vi "fireEventSendRefs.vi"(8 "error in (no error)":errorcluster, 10 "objectRefsMain":T1, 11 "sendRefs":refnum<user-event>) -> (0 "error out":errorcluster)   [LabVIEW 2017, in "User Event - Stop.lvlib"]
doc: "Send the Stop event to stop the Event Handling Loop."
uses:
  User Event - Stop.lvlib
  Controls/objectRefsMain.ctl
  sendRefs.ctl
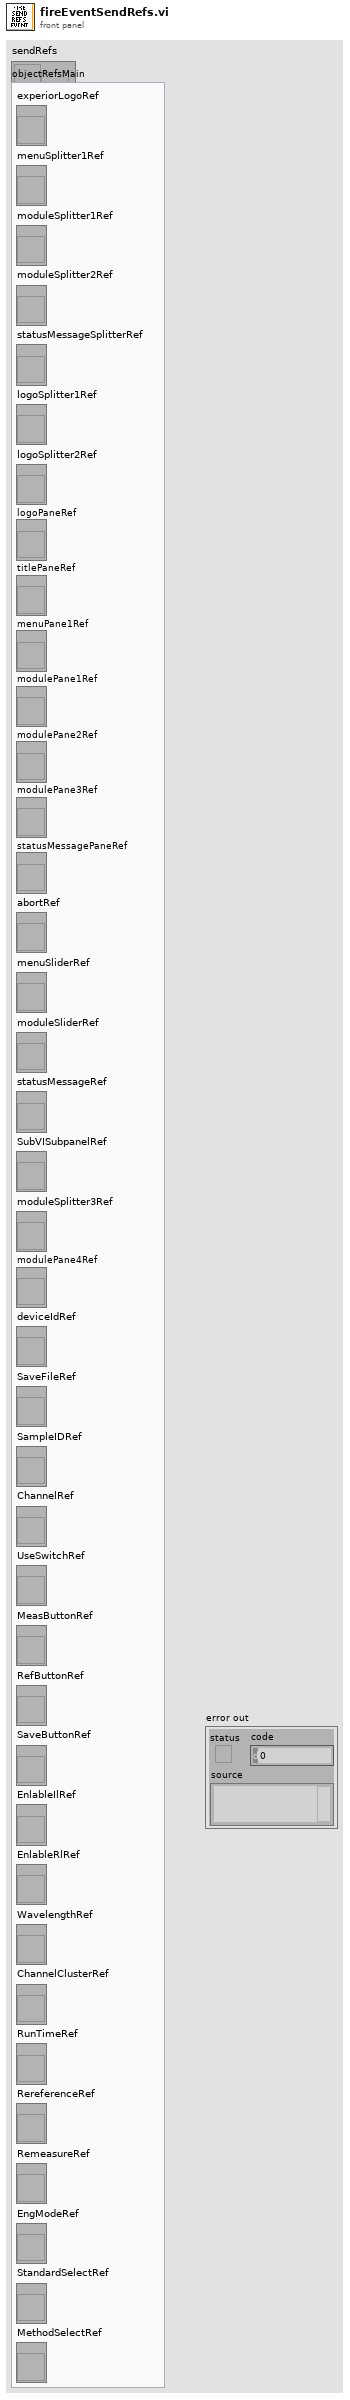
[diagram p1: front panel]
types:
  T1 = typedef "objectRefsMain.ctl" = cluster{"experiorLogoRef":refnum<vi>, "menuSplitter1Ref":refnum<vi>, "moduleSplitter1Ref":refnum<vi>, "moduleSplitter2Ref":refnum<vi>, "statusMessageSplitterRef":refnum<vi>, "logoSplitter1Ref":refnum<vi>, "logoSplitter2Ref":refnum<vi>, "logoPaneRef":refnum<vi>, "titlePaneRef":refnum<vi>, "menuPane1Ref":refnum<vi>, "modulePane1Ref":refnum<vi>, "modulePane2Ref":refnum<vi>, "modulePane3Ref":refnum<vi>, "statusMessagePaneRef":refnum<vi>, "abortRef":refnum<vi>, "menuSliderRef":refnum<vi>, "moduleSliderRef":refnum<vi>, "statusMessageRef":refnum<vi>, "SubVISubpanelRef":refnum<vi>, "moduleSplitter3Ref":refnum<vi>, "modulePane4Ref":refnum<vi>, "deviceIdRef":refnum<vi>, "SaveFileRef":refnum<vi>, "SampleIDRef":refnum<vi>, "ChannelRef":refnum<vi>, "UseSwitchRef":refnum<vi>, "MeasButtonRef":refnum<vi>, "RefButtonRef":refnum<vi>, "SaveButtonRef":refnum<vi>, "EnlableIlRef":refnum<vi>, "EnlableRlRef":refnum<vi>, "WavelengthRef":refnum<vi>, "ChannelClusterRef":refnum<vi>, "RunTimeRef":refnum<vi>, "RereferenceRef":refnum<vi>, "RemeasureRef":refnum<vi>, "EngModeRef":refnum<vi>, "StandardSelectRef":refnum<vi>, "MethodSelectRef":refnum<vi>}
  T2 = typedef "User Event - Stop.lvlib/sendRefs.ctl" = cluster{"objectRefsMain":T1}
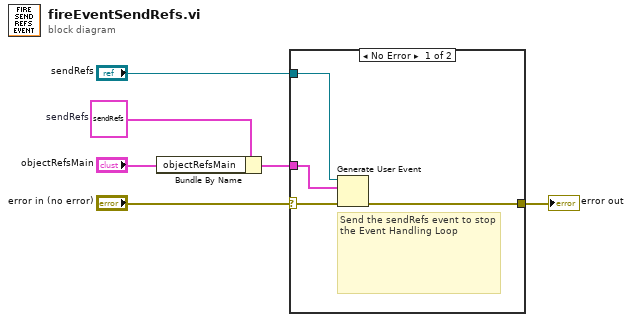
[diagram p0: block diagram]
diagram:
  w1 = T2 {"objectRefsMain"={"experiorLogoRef"=refnum, "menuSplitter1Ref"=refnum, "moduleSplitter1Ref"=refnum, "moduleSplitter2Ref"=refnum, "statusMessageSplitterRef"=refnum, "logoSplitter1Ref"=refnum, "logoSplitter2Ref"=refnum, "logoPaneRef"=refnum, "titlePaneRef"=refnum, "menuPane1Ref"=refnum, "modulePane1Ref"=refnum, "modulePane2Ref"=refnum, "modulePane3Ref"=refnum, "statusMessagePaneRef"=refnum, "abortRef"=refnum, "menuSliderRef"=refnum, "moduleSliderRef"=refnum, "statusMessageRef"=refnum, "SubVISubpanelRef"=refnum, "moduleSplitter3Ref"=refnum, "modulePane4Ref"=refnum, "deviceIdRef"=refnum, "SaveFileRef"=refnum, "SampleIDRef"=refnum, "ChannelRef"=refnum, "UseSwitchRef"=refnum, "MeasButtonRef"=refnum, "RefButtonRef"=refnum, "SaveButtonRef"=refnum, "EnlableIlRef"=refnum, "EnlableRlRef"=refnum, "WavelengthRef"=refnum, "ChannelClusterRef"=refnum, "RunTimeRef"=refnum, "RereferenceRef"=refnum, "RemeasureRef"=refnum, "EngModeRef"=refnum, "StandardSelectRef"=refnum, "MethodSelectRef"=refnum}}  # sendRefs
  n1 = Bundle By Name(cluster=w1, "objectRefsMain"="objectRefsMain") -> (w2:T2)
  n2 = case shown="No Error" "error in (no error)" {
    selector: "error in (no error)" -> [w8 w11]
    tunnel: [w10 w11] -> w6
    tunnel: "sendRefs" -> [w9 _]
    tunnel: w2 -> [w7 _]
    frame No Error {
      # "Send the sendRefs event to stop the Event Handling Loop"
      n3 = Generate User Event(user event=w9, event data cluster=w7, error in=w8) -> (error out=w10:errorcluster)  [unwired: 1 in, 1 out]
    }
    frame Error {
    }
  }
  "error out" <- w6
